vi "Data Record.vi"(8 "TD1 Pressure":dbl, 9 "TD0 Pressure":dbl, 10 "Timestamp":u32, 11 "file ref in":refnum<file>) -> (1 "Record Time":dbl, 3 "refnum out":refnum<file>)   [LabVIEW 2015]
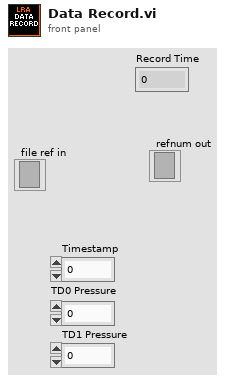
[diagram p1: front panel]
types:
  T1 = enum16{"open", "replace", "create", "open or create", "replace or create", "replace or create with confirmation"}
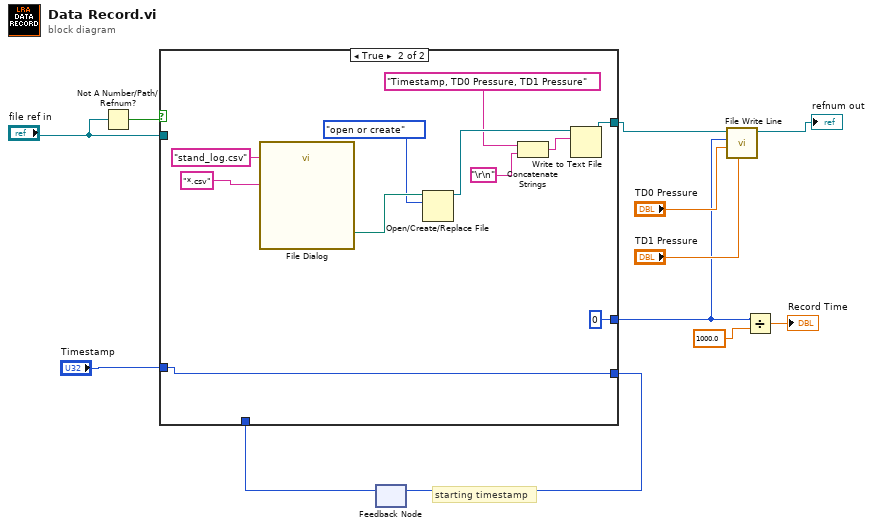
[diagram p0: block diagram]
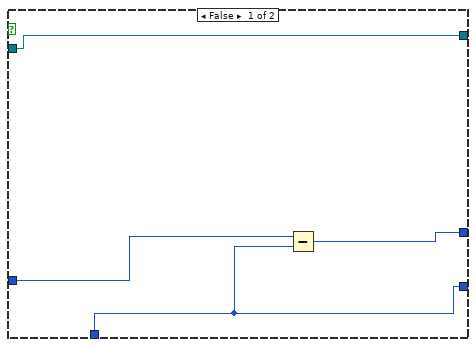
[diagram p2: hidden frame]
diagram:
  # "starting timestamp"
  n1 = Not A Number/Path/Refnum?(number/path/refnum="file ref in") -> (NaN/Path/Refnum?=w7:bool)
  n2 = feedback #1() -> (w4:u32)  [unwired: 1 in]
  n3 = case shown="True" w7 {
    tunnel: "file ref in" -> [w16 _]
    tunnel: [w16 w22] -> w10
    tunnel: "Timestamp" -> [w15 w21]
    tunnel: [w13 w21] -> w5
    tunnel: w4 -> [w13 _]
    tunnel: [w14 u32 0] -> w3
    frame False {
      n4 = Subtract(x=w15, y=w13) -> (x-y=w14:u32)
    }
    frame True {
      n5 = call "File Dialog"("default name"="stand_log.csv", "pattern label"="*.csv") -> ("selected path"=w25:path)  [unwired: 10 in, 3 out]
      n6 = Open/Create/Replace File(file path (use dialog)=w25, operation (0:open)=T1."open or create") -> (refnum out=w23:refnum<file>)  [unwired: 4 in, 2 out]
      n7 = Concatenate Strings("Timestamp, TD0 Pressure, TD1 Pressure" ("text"), "\r\n") -> (w17:string)
      n8 = Write to Text File(file (use dialog)=w23, text=w17) -> (refnum out=w22:refnum<file>)  [unwired: 2 in, 2 out]
    }
  }
  n9 = feedback-in #1(w5) -> ()
  n10 = call "File Write Line.vi"("TD1 Pressure"="TD1 Pressure", "TD0 Pressure"="TD0 Pressure", "Timestamp"=w3, "file in"=w10) -> ("Byte Stream File out"=→"refnum out":refnum<file>)  [unwired: 7 in]
  n11 = Divide(x=w3, y=1000.0) -> (x/y=→"Record Time":dbl)
